vi "DriveBalance.vi"(2 "Parameter String":string="near", 3 "Reinit":bool) -> (0 "Error Out":errorcluster, 1 "Increment":bool)   [LabVIEW 2020]
doc: "The swerve drive base will translate in the field-centric X direction until it reaches the CHARGING STATION. Then it will move up the ramp and balance using the pitch feedback from the IMU.\n\nParameters:\n1. \"near\" or \"far\" to indicate which side the robot is coming from in relation to the driver station"
uses:
  fecc16b4-9204-47e7-b057-41e41d998ae7.vi
  0fe48bd2-3b49-4c8c-82c6-f24528f2b59d.vi
  9c209fce-094d-437e-8f6c-1b0f354aa5a3.vi
  3ab4cadb-8a01-4273-86b8-f239e16545bb.vi
  SafeParser_String.vi
  GlobalDriverStationData.vi
  GlobalDriverStationCommands.vi
  GlobalPoseAndTargeting.vi
panel:
  in  "Movement stopped threshold":dbl=2.0
  in  "Balancing Kp":dbl=0.002
  in  "Power Integration per Loop":dbl=0.001 format="%#_13g"
  in  "Power to Drive to Ramp":dbl=0.3 format="%#_13g"
  in  "Gravity Feed-Froward":dbl=0.15
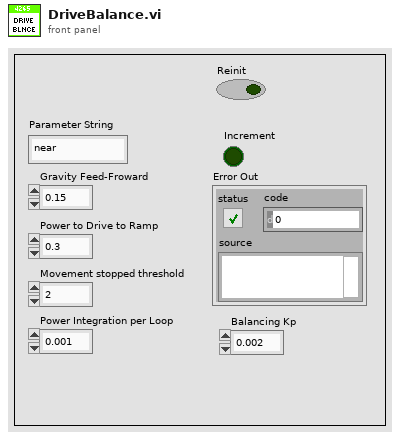
[diagram p1: front panel]
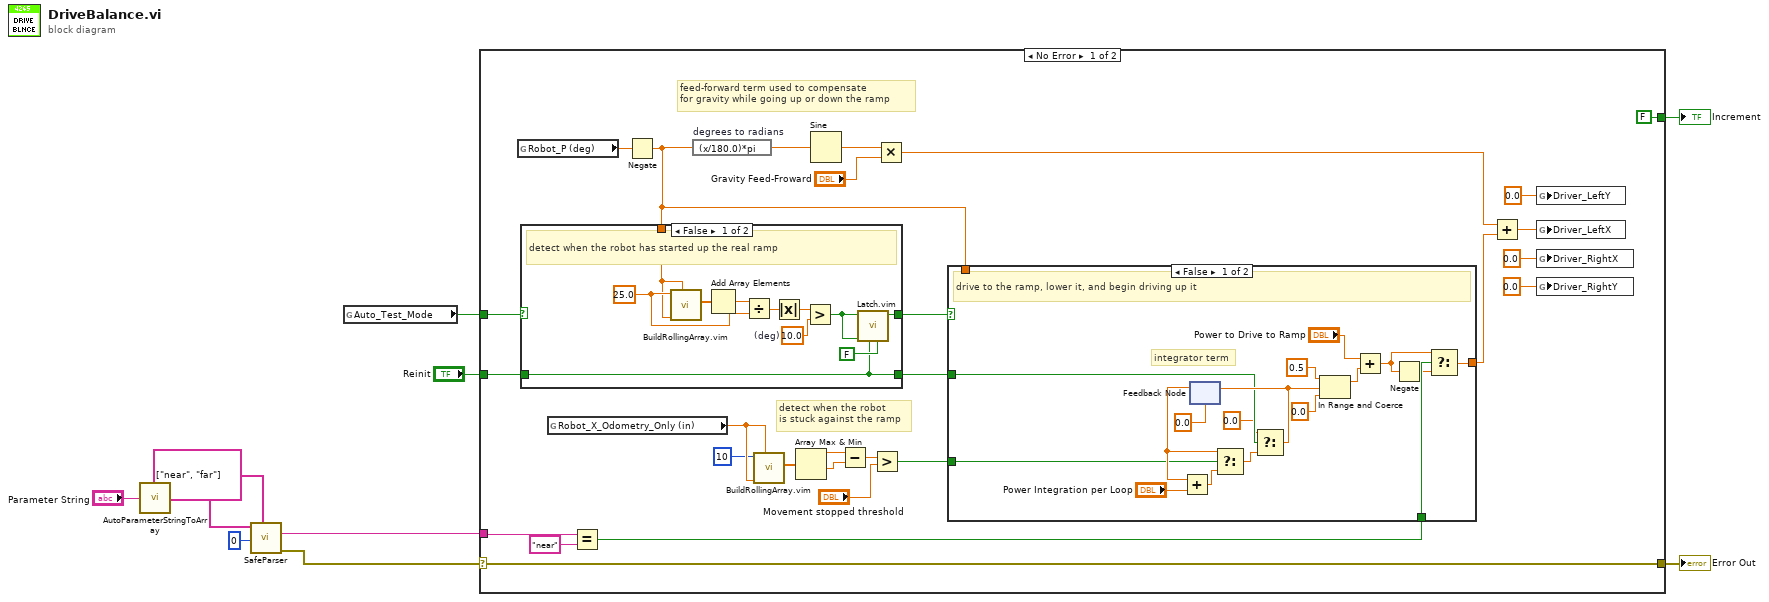
[diagram p0: block diagram]
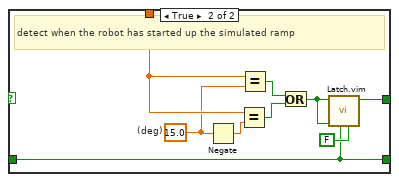
[diagram p2: hidden frame]
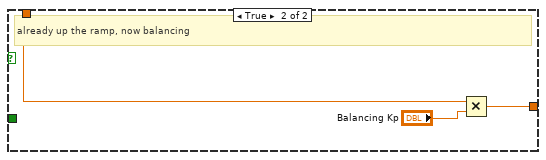
[diagram p3: hidden frame]
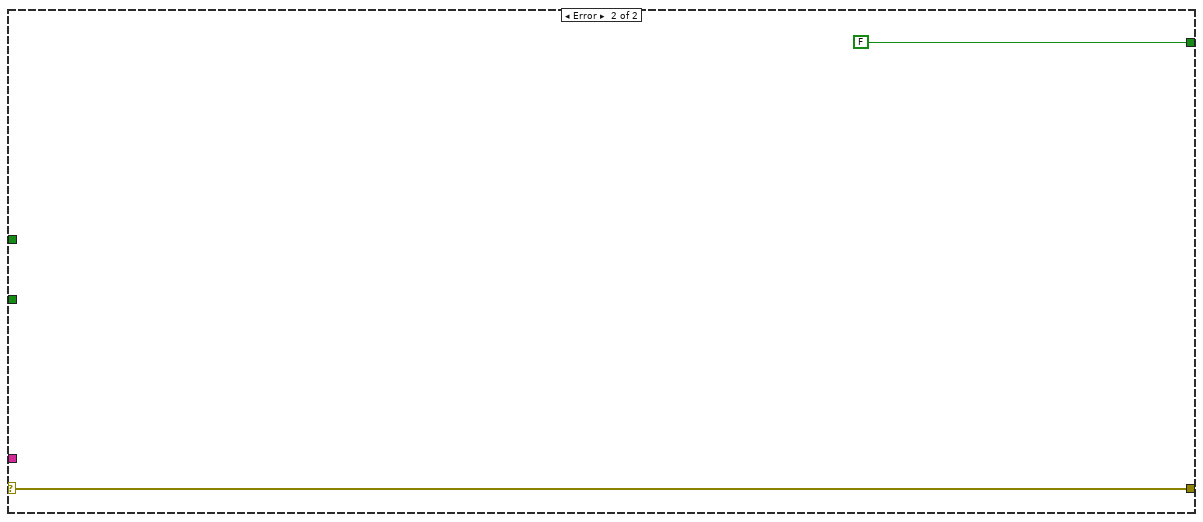
[diagram p4: hidden frame]
diagram:
  n1 = call "AutoParameterStringToArray.vi"("Parameter String"="Parameter String") -> ("Parsed Parameters"=w7:string[])
  n2 = call-poly "SafeParser.vi"("Allowed Values"=string[] ["near", "far"], "Array Index"=0 ("Parameter Index"), "String Array"=w7) -> ("Error Out"=w2:errorcluster, "Typecast Value"=w6:string)  [unwired: 7 in]
  n3 = global read "GlobalDriverStationData.vi" "Auto_Test_Mode"() -> (w1:bool)
  n4 = case shown="No Error" w2 {
    selector: w2 -> [w38 w80]
    tunnel: [FALSE FALSE] -> w4
    tunnel: "Reinit" -> [w21 _]
    tunnel: [w38 w80] -> w9
    tunnel: w6 -> [w35 _]
    tunnel: w1 -> [w19 _]
    frame No Error {
      # "detect when the robot\nis stuck against the ramp"
      # "feed-forward term used to compensate\nfor gravity while going up or down the ramp"
      n5 = global read "GlobalPoseAndTargeting.vi" "Robot_P (deg)"() -> (w36:dbl)
      n6 = global read "GlobalPoseAndTargeting.vi" "Robot_X_Odometry_Only (in)"() -> (w18:dbl)
      n7 = Equal?(x=w35, y="near") -> (x = y?=w23:bool)
      n8 = Negate(x=w36) -> (-x=w22:dbl)
      n9 = case shown="False" w19 {
        tunnel: [w42 w56] -> w24
        tunnel: w22 -> [w41 w55]
        tunnel: w21 -> [w39 w57]
        tunnel: [w39 w57] -> w20
        frame False {
          w45 = 10.0  # (deg)
          w47 = 25.0 ("Number of Elements")
          # "detect when the robot has started up the real ramp"
          n10 = call "BuildRollingArray.vim"("New Value"=w41, "Initial Value"=w41, "Number of Elements"=w47) -> ("Current Array"=w49:dbl[])  [unwired: 8 in]
          n11 = Add Array Elements(numeric array=w49) -> (sum=w48:dbl)
          n12 = Divide(x=w48, y=w47) -> (x/y=w46:dbl)
          n13 = Absolute Value(x=w46) -> (abs(x)=w40:dbl)
          n14 = Greater?(x=w40, y=w45) -> (0:w43:bool)
          n15 = call "Latch.vim"("Default Value"=FALSE, "Reset"=w39, "Latch Signal"=w43, "Latch Value"=w43) -> ("Latched"=w42:bool)  [unwired: 7 in]
        }
        frame True {
          w50 = 15.0  # (deg)
          # "detect when the robot has started up the simulated ramp"
          n16 = Negate(x=w50) -> (-x=w51:dbl)
          n17 = Equal?(x=w55, y=w51) -> (x = y?=w53:bool)
          n18 = Equal?(x=w55, y=w50) -> (x = y?=w54:bool)
          n19 = Or(x=w54, y=w53) -> (x .or. y?=w52:bool)
          n20 = call "Latch.vim"("Default Value"=FALSE, "Reset"=w57, "Latch Signal"=w52, "Latch Value"=w52) -> ("Latched"=w56:bool)  [unwired: 7 in]
        }
      }
      n21 = expression code="(x/180.0)*pi" "degrees to radians"(w22) -> (w31:dbl)
      n22 = call "BuildRollingArray.vim"("New Value"=w18, "Initial Value"=w18, "Number of Elements"=10) -> ("Current Array"=w17:dbl[])  [unwired: 8 in]
      n23 = Array Max & Min(array=w17) -> (max value=w16:dbl, min value=w15:dbl)  [unwired: 2 out]
      n24 = Sine(x=w31) -> (sin(x)=w32:dbl)
      n25 = Subtract(x=w16, y=w15) -> (x-y=w14:dbl)
      n26 = Greater?(x=w14, y="Movement stopped threshold") -> (0:w12:bool)
      n27 = Multiply(x=w32, y="Gravity Feed-Froward") -> (x*y=w33:dbl)
      n28 = case shown="False" w24 {
        tunnel: [w60 w77] -> w30
        tunnel: w22 -> [_ w76]
        tunnel: w23 -> [w71 _]
        tunnel: w20 -> [w65 _]
        tunnel: w12 -> [w59 _]
        frame False {
          # "integrator term"
          # "drive to the ramp, lower it, and begin driving up it"
          n29 = feedback #1(0.0) -> (w73:dbl)
          n30 = Add(x=w73, y="Power Integration per Loop") -> (x+y=w74:dbl)
          n31 = Select(t=w73, s=w59, f=w74) -> (s? t:f=w68:dbl)
          n32 = Select(t=0.0, s=w65, f=w68) -> (s? t:f=w66:dbl)
          n33 = feedback-in #1(w66) -> ()
          n34 = In Range and Coerce(upper limit=0.5, x=w66, lower limit=0.0) -> (coerced(x)=w67:dbl)  [unwired: 1 out]
          n35 = Add(x="Power to Drive to Ramp", y=w67) -> (x+y=w62:dbl)
          n36 = Negate(x=w62) -> (-x=w61:dbl)
          n37 = Select(t=w62, s=w71, f=w61) -> (s? t:f=w60:dbl)
        }
        frame True {
          # "already up the ramp, now balancing"
          n38 = Multiply(x=w76, y="Balancing Kp") -> (x*y=w77:dbl)
        }
      }
      n39 = Add(x=w33, y=w30) -> (x+y=w26:dbl)
      n40 = global write "GlobalDriverStationCommands.vi" "Driver_LeftY"(0.0 ("Driver_LeftY")) -> ()
      n41 = global write "GlobalDriverStationCommands.vi" "Driver_LeftX"(w26) -> ()
      n42 = global write "GlobalDriverStationCommands.vi" "Driver_RightX"(0.0 ("Driver_RightX")) -> ()
      n43 = global write "GlobalDriverStationCommands.vi" "Driver_RightY"(0.0 ("Driver_RightX")) -> ()
    }
    frame Error {
    }
  }
  "Increment" <- w4
  "Error Out" <- w9
